vi "PH_Beckhoff_PPMA-Rods.constructor.vi"(0 "name":string, 2 "data in":string, 5 "error in(no error)":errorcluster) -> (14 "i ref out":refnum<vi>, 16 "data out":string, 19 "error out":errorcluster)   [LabVIEW 2014, in "PH_Beckhoff_PPMA-Rods.lvlib"]
doc: "This is the constructor of a class.\n\nLicense Agreement for this software:\n\nCopyright (C)\nGesellschaft für Schwerionenforschung, GSI\nPlanckstr. 1\n64291 Darmstadt\nGermany\n\nContact: D.Beck@gsi.de \n\nThis program is free software; you can redistribute it and/or modify it under the terms of the \nGNU General Public License as published by the Free Software Foundation; either version 2 of \nthe license, or (at your option) any later version.\n\nThis program is distributed in the hope that it will be useful, but WITHOUT ANY WARRANTY; \nwithout even the implied warranty of MERCHANTABILITY or FITNESS FOR A PARTICULAR PURPOSE. See the GNU General License for more details (http://www.gnu.org).\n\nGesellschaft für Schwerionenforschung, GSI\nPlanckstr. 1, 64291 Darmstadt, Germany\nFor all questions and ideas contact: M.Richter@gsi.de, H.Brand@gsi.de or D.Beck@gsi.de.\nLast update: 16-JUN-2004"
uses:
  PH_Beckhoff_PPMA-Rods.lvlib
  CS_Core/CSSystem/CSSystemLib/CSSystemLib.lvlib
  PH_Beckhoff/PH_Beckhoff.lvlib
  PH_Basics/PH_Class/PH_Class.lvlib
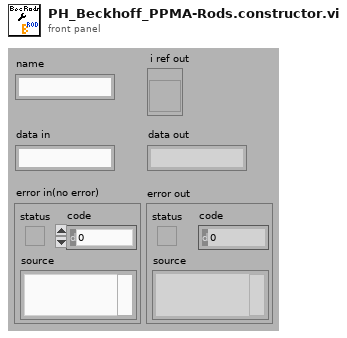
[diagram p1: front panel]
types:
  T1 = enum16{"SetAttribute", "GetAttribute", "CreateAttribute", "DestroyAttribute", "DestroyAllAtributes"}
  T2 = typedef "PH_Beckhoff.lvlib/PH_Beckhoff.constructor Data in.ctl" = cluster{"Default Values":T3, "Description":string, "Hardware configured?":bool, "Activate Change Manager?":bool, "Difference to handle an analog input as change":u32}
  T3 = typedef "PH_Beckhoff.lvlib/PH_Beckhoff.Values.ctl" = cluster{"Sonderklemmen Inputs":T4, "Analog Inputs":T5, "Analog Outputs":T7, "Digital Inputs":T8, "Digital Outputs":T9}
  T4 = typedef "PH_Beckhoff.lvlib/PH_Beckhoff.Sonderklemmen Inputs.ctl" = cluster{"Total Length":u32, "Name":string, "Value":u64, "Quality":bool, "Service ID":i32, "Offset":u32, "Length":u32}[]
  T5 = typedef "PH_Beckhoff.lvlib/PH_Beckhoff.Analog Inputs.ctl" = cluster{"Name":string, "Value":u32, "Quality":bool, "Service ID":i32, "Sca Type":T6}[]
  T6 = typedef "PH_Beckhoff.lvlib/PH_Beckhoff.Scaling Type.ctl" = enum16{"none", "0 ... 15 Bit -> 0 ... 5", "0 ... 15 Bit -> 0 ... 10", "0 ... 15 Bit -> 0 ... 25", "0 ... 15 Bit -> 4 ... 20", "0 ... 15 Bit -> 0 ... 1", "0 ... 15 Bit -> 0 ... 20000", "0 ... 15 Bit -> 0 ... 24000"}
  T7 = typedef "PH_Beckhoff.lvlib/PH_Beckhoff.Analog Outputs.ctl" = cluster{"Name":string, "Value":u32, "Quality":bool, "Wanted Value":u32, "Service ID":i32, "Sca Type":T6}[]
  T8 = typedef "PH_Beckhoff.lvlib/PH_Beckhoff.Digital Inputs.ctl" = cluster{"Name":string, "Value":bool, "Quality":bool, "Service ID":i32, "inverted?":bool}[]
  T9 = typedef "PH_Beckhoff.lvlib/PH_Beckhoff.Digital Outputs.ctl" = cluster{"Name":string, "Value":bool, "Quality":bool, "Wanted Value":bool, "Service ID":i32, "inverted?":bool}[]
  T10 = typedef "PH_Beckhoff_PPMA-Rods.lvlib/PH_Beckhoff_PPMA-Rods.i attribute.ctl" = cluster{"Input Up GUI Refs":refnum<vi>[], "Output GUI Refs":cluster{"Rod A up":refnum<vi>, "Rod B up":refnum<vi>, "Warnlamp orange":refnum<vi>, "Warnlamp green":refnum<vi>}, "States":cluster{"GUI Ref":refnum<vi>, "Status":T11, "Service ID":i32}[], "Input GUI Refs":cluster{"earth ok":refnum<vi>, "door locked K1":refnum<vi>, "door locked K2":refnum<vi>, "valve closed":refnum<vi>}}
  T11 = typedef "PH_StatusHandler.lvlib/PH_StatusHandler.Status.ctl" = i16
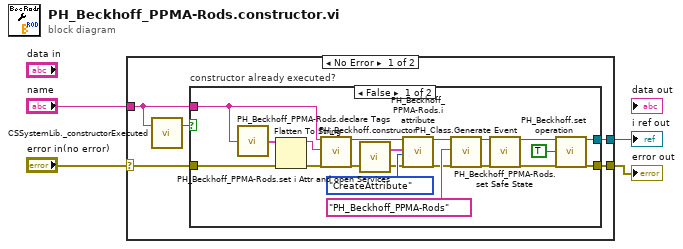
[diagram p0: block diagram]
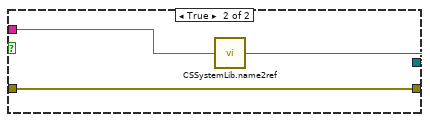
[diagram p2: hidden frame]
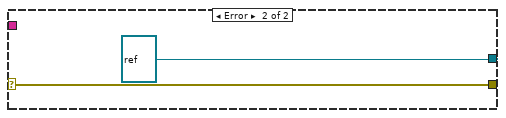
[diagram p3: hidden frame]
diagram:
  n1 = case shown="No Error" "error in(no error)" {
    selector: "error in(no error)" -> [w7 w34]
    tunnel: "name" -> [w6 _]
    tunnel: [w9 refnum<vi> refnum ("obj refnum")] -> w3
    tunnel: [w8 w34] -> w2
    frame No Error {
      n2 = call "CSSystemLib._constructorExecuted.vi"("name"=w6) -> ("constructor executed?"=w5:bool)  [unwired: 18 in]
      n3 = case "constructor already executed?" shown="False" w5 {
        tunnel: [w21 w31] -> w9
        tunnel: [w22 w30] -> w8
        tunnel: w7 -> [w10 w30]
        tunnel: w6 -> [w11 w32]
        frame False {
          n4 = call "PH_Beckhoff_PPMA-Rods.declare Tags.vi"("Instance Name"=w11) -> ("Data in cluster"=w27:T2)
          n5 = Flatten To String(anything=w27, error in (no error)=w10) -> (data string=w28:string, error out=w29:errorcluster)  [unwired: 2 in, 1 out]
          n6 = call "PH_Beckhoff.constructor.vi"("name"=w11, "data in"=w28, "error in(no error)"=w29) -> ("i ref out"=w13:refnum<vi>, "error out"=w20:errorcluster)  [unwired: 14 in, 1 out]
          n7 = call "PH_Beckhoff_PPMA-Rods.set i Attr and open Services.vi"("error in"=w20) -> ("error out"=w25:errorcluster, "i Attr"=w24:T10)  [unwired: 1 in]
          n8 = call "PH_Beckhoff_PPMA-Rods.i attribute.vi"("VI Refnum"=w13, "CLASS.i attribute"=w24, "Action"=T1."CreateAttribute", "error in (no error)"=w25) -> ("VI Refnum out"=w12:refnum<vi>, "error out"=w16:errorcluster)  [unwired: 13 in, 1 out]
          n9 = call "PH_Class.Generate Event.vi"("i ref in"=w12, "Class"="PH_Beckhoff_PPMA-Rods", "error in (no error)"=w16) -> ("i ref out"=w14:refnum<vi>, "error out"=w15:errorcluster)  [unwired: 15 in]
          n10 = call "PH_Beckhoff_PPMA-Rods.set Safe State.vi"("i ref in"=w14, "error in"=w15) -> ("i ref out"=w17:refnum<vi>, "error out"=w18:errorcluster)  [unwired: 16 in]
          n11 = call "PH_Beckhoff.set operation.vi"("VI in"=w17, "operation?"=TRUE, "error in (no error)"=w18) -> ("VI out"=w21:refnum<vi>, "error out"=w22:errorcluster)  [unwired: 15 in]
        }
        frame True {
          n12 = call "CSSystemLib.name2ref.vi"("name"=w32) -> ("obj refnum"=w31:refnum<vi>)
        }
      }
    }
    frame Error {
    }
  }
  "i ref out" <- w3
  "error out" <- w2
